vi "myRIO_BRig_Host_formatData_getHeaders_dataBlock.vi"() -> (3 "output_stringArray_dataBlock":string[](array[string]))   [LabVIEW 2014]
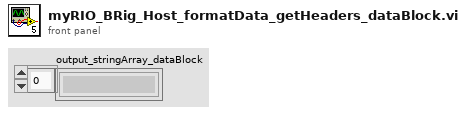
[diagram p1: front panel]
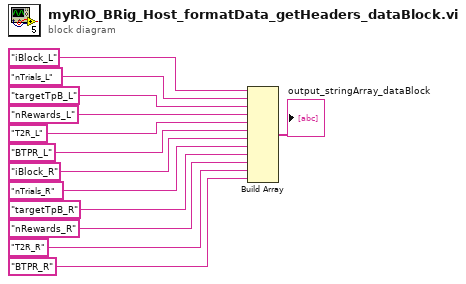
[diagram p0: block diagram]
diagram:
  n1 = Build Array("iBlock_L", "nTrials_L", "targetTpB_L", "nRewards_L", "T2R_L", "BTPR_L", "iBlock_R", "nTrials_R", "targetTpB_R", "nRewards_R", "T2R_R", "BTPR_R") -> (→"output_stringArray_dataBlock":string[])
